vi "Close.vi"(8 "error in":errorcluster, 11 "Power Supply In":refnum<class "Power Supply.lvclass">) -> (0 "error out":errorcluster, 3 "Power Supply Out":refnum<class "Power Supply.lvclass">)   [LabVIEW 2023, in "Power Supply.lvclass"]
uses:
  Power Supply.lvclass
  Power Supply.lvclass/Power Supply.ctl
  Low Level Capabilities/Output Enable/Output Enable.lvclass
  Low Level Capabilities/OnOff/OnOff.lvclass
  Low Level Capabilities/Error/Error.lvclass
  Low Level Capabilities/Power/Power Setpoint/Power Setpoint.lvclass
  Low Level Capabilities/Power/Power Actual Value/Power Actual Value.lvclass
  Low Level Capabilities/Power/Power Limit/Power Limit.lvclass
  Low Level Capabilities/Voltage/Voltage Limit/Voltage Limit.lvclass
  Low Level Capabilities/Control Mode/Control Mode.lvclass
  Low Level Capabilities/Error Channels/Error Channels.lvclass
  Low Level Capabilities/Current/Current Limit/Current Limit.lvclass
  Low Level Capabilities/Current/Current Actual Value/Current Actual Value.lvclass
  Low Level Capabilities/Current/Current Setpoint/Current Setpoint.lvclass
  Low Level Capabilities/Voltage/Voltage Actual Value/Voltage Actual Value.lvclass
  Low Level Capabilities/Voltage/Voltage Setpoint/Voltage Setpoint.lvclass
  Low Level Capabilities/Voltage/Voltage Gradient/Voltage Gradient.lvclass
  Low Level Capabilities/Power/Power Gradient/Power Gradient.lvclass
  Low Level Capabilities/Current/Current Gradient/Current Gradient.lvclass
panel:
  in  "not in use":string="Setpoint.ch%d.SP"
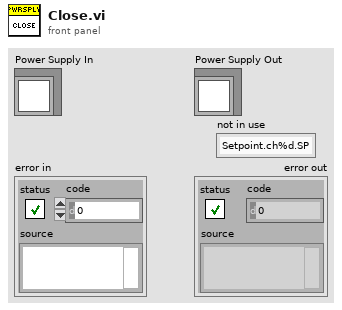
[diagram p1: front panel]
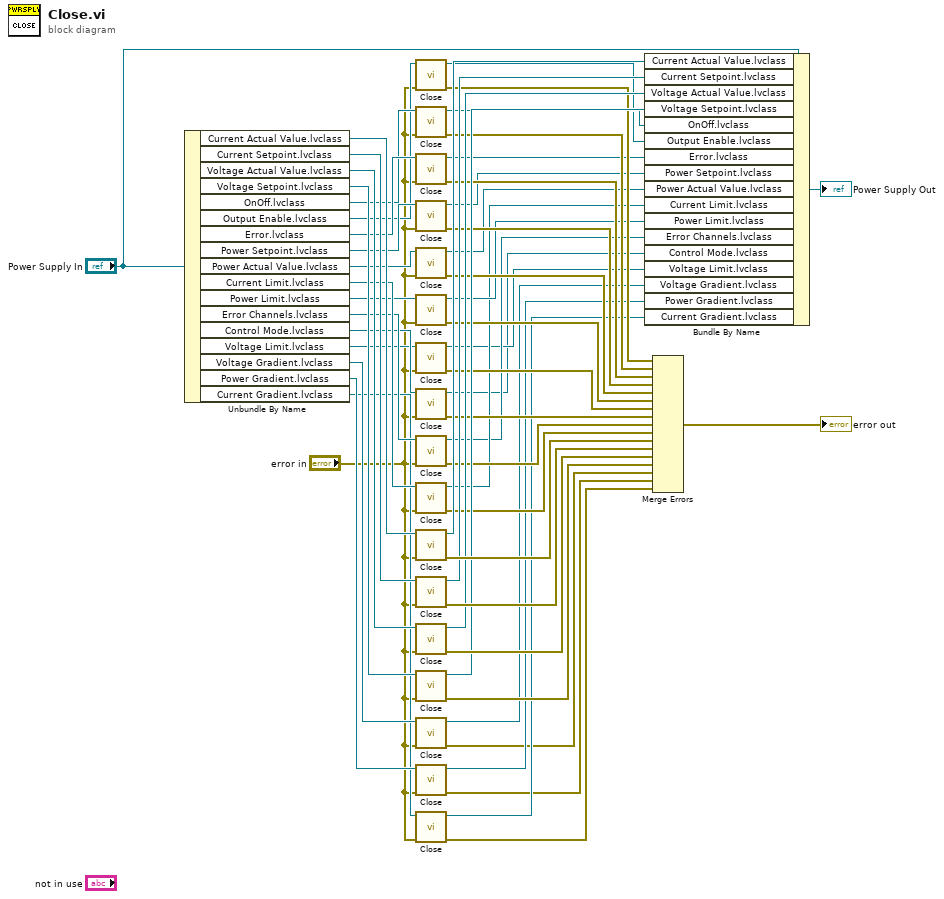
[diagram p0: block diagram]
diagram:
  n1 = Unbundle By Name("Power Supply In") -> ("Current Actual Value.lvclass"=w50:refnum<class "Current Actual Value.lvclass">, "Current Setpoint.lvclass"=w49:refnum<class "Current Setpoint.lvclass">, "Voltage Actual Value.lvclass"=w47:refnum<class "Voltage Actual Value.lvclass">, "Voltage Setpoint.lvclass"=w46:refnum<class "Voltage Setpoint.lvclass">, "OnOff.lvclass"=w27:refnum<class "OnOff.lvclass">, "Output Enable.lvclass"=w24:refnum<class "Output Enable.lvclass">, "Error.lvclass"=w28:refnum<class "Error.lvclass">, "Power Setpoint.lvclass"=w30:refnum<class "Power Setpoint.lvclass">, "Power Actual Value.lvclass"=w33:refnum<class "Power Actual Value.lvclass">, "Current Limit.lvclass"=w43:refnum<class "Current Limit.lvclass">, "Power Limit.lvclass"=w35:refnum<class "Power Limit.lvclass">, "Error Channels.lvclass"=w41:refnum<class "Error Channels.lvclass">, "Control Mode.lvclass"=w39:refnum<class "Control Mode.lvclass">, "Voltage Limit.lvclass"=w36:refnum<class "Voltage Limit.lvclass">, "Voltage Gradient.lvclass"=w10:refnum<class "Voltage Gradient.lvclass">, "Power Gradient.lvclass"=w9:refnum<class "Power Gradient.lvclass">, "Current Gradient.lvclass"=w8:refnum<class "Current Gradient.lvclass">)
  n2 = call-dynamic "Close.vi"("error in"="error in", "Output Enable in"=w24) -> ("error out"=w25:errorcluster, "Output Enable out"=w22:refnum<class "Output Enable.lvclass">)  [unwired: 8 in]
  n3 = call-dynamic "Close.vi"("error in"="error in", "OnOff in"=w27) -> ("error out"=w26:errorcluster, "OnOff out"=w23:refnum<class "OnOff.lvclass">)  [unwired: 8 in]
  n4 = call-dynamic "Close.vi"("error in"="error in", "Error in"=w28) -> ("error out"=w29:errorcluster, "Error out"=w21:refnum<class "Error.lvclass">)  [unwired: 8 in]
  n5 = call-dynamic "Close.vi"("error in"="error in", "Power Setpoint in"=w30) -> ("error out"=w31:errorcluster, "Power Setpoint out"=w20:refnum<class "Power Setpoint.lvclass">)  [unwired: 8 in]
  n6 = call-dynamic "Close.vi"("error in"="error in", "Power Actual Value in"=w33) -> ("error out"=w32:errorcluster, "Power Actual Value out"=w19:refnum<class "Power Actual Value.lvclass">)  [unwired: 8 in]
  n7 = call-dynamic "Close.vi"("error in"="error in", "Power Limit in"=w35) -> ("error out"=w34:errorcluster, "Power Limit out"=w18:refnum<class "Power Limit.lvclass">)  [unwired: 8 in]
  n8 = call-dynamic "Close.vi"("error in"="error in", "Voltage Limit in"=w36) -> ("error out"=w37:errorcluster, "Voltage Limit out"=w15:refnum<class "Voltage Limit.lvclass">)  [unwired: 8 in]
  n9 = call-dynamic "Close.vi"("error in"="error in", "Control Mode in"=w39) -> ("error out"=w38:errorcluster, "Control Mode out"=w14:refnum<class "Control Mode.lvclass">)  [unwired: 8 in]
  n10 = call-dynamic "Close.vi"("error in"="error in", "Error Channels in"=w41) -> ("error out"=w40:errorcluster, "Error Channels out"=w16:refnum<class "Error Channels.lvclass">)  [unwired: 8 in]
  n11 = call-dynamic "Close.vi"("error in"="error in", "Current Limit in"=w43) -> ("error out"=w42:errorcluster, "Current Limit out"=w17:refnum<class "Current Limit.lvclass">)  [unwired: 8 in]
  n12 = call-dynamic "Close.vi"("error in"="error in", "Current Actual Value in"=w50) -> ("error out"=w54:errorcluster, "Current Actual Value out"=w51:refnum<class "Current Actual Value.lvclass">)  [unwired: 8 in]
  n13 = call-dynamic "Close.vi"("error in"="error in", "Current Setpoint in"=w49) -> ("error out"=w55:errorcluster, "Current Setpoint out"=w48:refnum<class "Current Setpoint.lvclass">)  [unwired: 8 in]
  n14 = call-dynamic "Close.vi"("error in"="error in", "Voltage Actual Value in"=w47) -> ("error out"=w53:errorcluster, "Voltage Actual Value out"=w45:refnum<class "Voltage Actual Value.lvclass">)  [unwired: 8 in]
  n15 = call-dynamic "Close.vi"("error in"="error in", "Voltage Setpoint in"=w46) -> ("error out"=w52:errorcluster, "Voltage Setpoint out"=w44:refnum<class "Voltage Setpoint.lvclass">)  [unwired: 8 in]
  n16 = call-dynamic "Close.vi"("error in"="error in", "Voltage Gradient in"=w10) -> ("error out"=w7:errorcluster, "Voltage Gradient out"=w13:refnum<class "Voltage Gradient.lvclass">)  [unwired: 8 in]
  n17 = call-dynamic "Close.vi"("error in"="error in", "Power Gradient in"=w9) -> ("error out"=w6:errorcluster, "Power Gradient out"=w12:refnum<class "Power Gradient.lvclass">)  [unwired: 8 in]
  n18 = call-dynamic "Close.vi"("error in"="error in", "Current Gradient in"=w8) -> ("error out"=w5:errorcluster, "Current Gradient out"=w11:refnum<class "Current Gradient.lvclass">)  [unwired: 8 in]
  n19 = Bundle By Name(cluster="Power Supply In", "Current Actual Value.lvclass"=w51, "Current Setpoint.lvclass"=w48, "Voltage Actual Value.lvclass"=w45, "Voltage Setpoint.lvclass"=w44, "OnOff.lvclass"=w23, "Output Enable.lvclass"=w22, "Error.lvclass"=w21, "Power Setpoint.lvclass"=w20, "Power Actual Value.lvclass"=w19, "Current Limit.lvclass"=w17, "Power Limit.lvclass"=w18, "Error Channels.lvclass"=w16, "Control Mode.lvclass"=w14, "Voltage Limit.lvclass"=w15, "Voltage Gradient.lvclass"=w13, "Power Gradient.lvclass"=w12, "Current Gradient.lvclass"=w11) -> (→"Power Supply Out":refnum<class "Power Supply.lvclass">)
  n20 = Merge Errors(w25, w26, w29, w31, w32, w34, w37, w38, w40, w42, w54, w55, w53, w52, w7, w6, w5) -> (→"error out":errorcluster)
